vi "DCPower_ConfigureInstrument_V2.vi"(0 "IVI Refnum in":refnum<k15>, 1 "current limit":dbl, 2 "Aperture Time":dbl, 3 "Measure Record Length":i32, 4 "Active Channels Input":bool[](array[boolean]), 5 "Channel Name Array":string[](array[string]), 7 "error in (no error)":errorcluster, 8 "Voltage Array Input":dbl[](array[numeric]), 10 "DCPowerInformationClusterArray_Input":T1(array[cluster])) -> (12 "Active Channels Indicator":bool[](array[boolean]), 14 "All Channel Numbers Array":string[](array[string]), 16 "Total Voltage Indicator Array":dbl[](array[numeric]), 17 "All Channels Numbers List":string, 18 "Active Channel Numbers String List":string, 19 "IVI Ref index":i32, 20 "IVI Refnum out":refnum<k15>, 21 "Active Channel Numbers Array":string[](array[string]), 22 "Active Channel Names Array":string[](array[string]), 23 "Active Channel Current Limit Array":dbl[](array[numeric]), 24 "Active Channel Measure Record Delta Time Array":dbl[](array[numeric]), 25 "Active Channel Voltage Array":dbl[](array[numeric]), 26 "IVI Ref Present?":bool, 27 "error out":errorcluster)   [LabVIEW 2019]
panel:
  in  "DCPowerInformationClusterArray_Input_":T2(array[cluster])
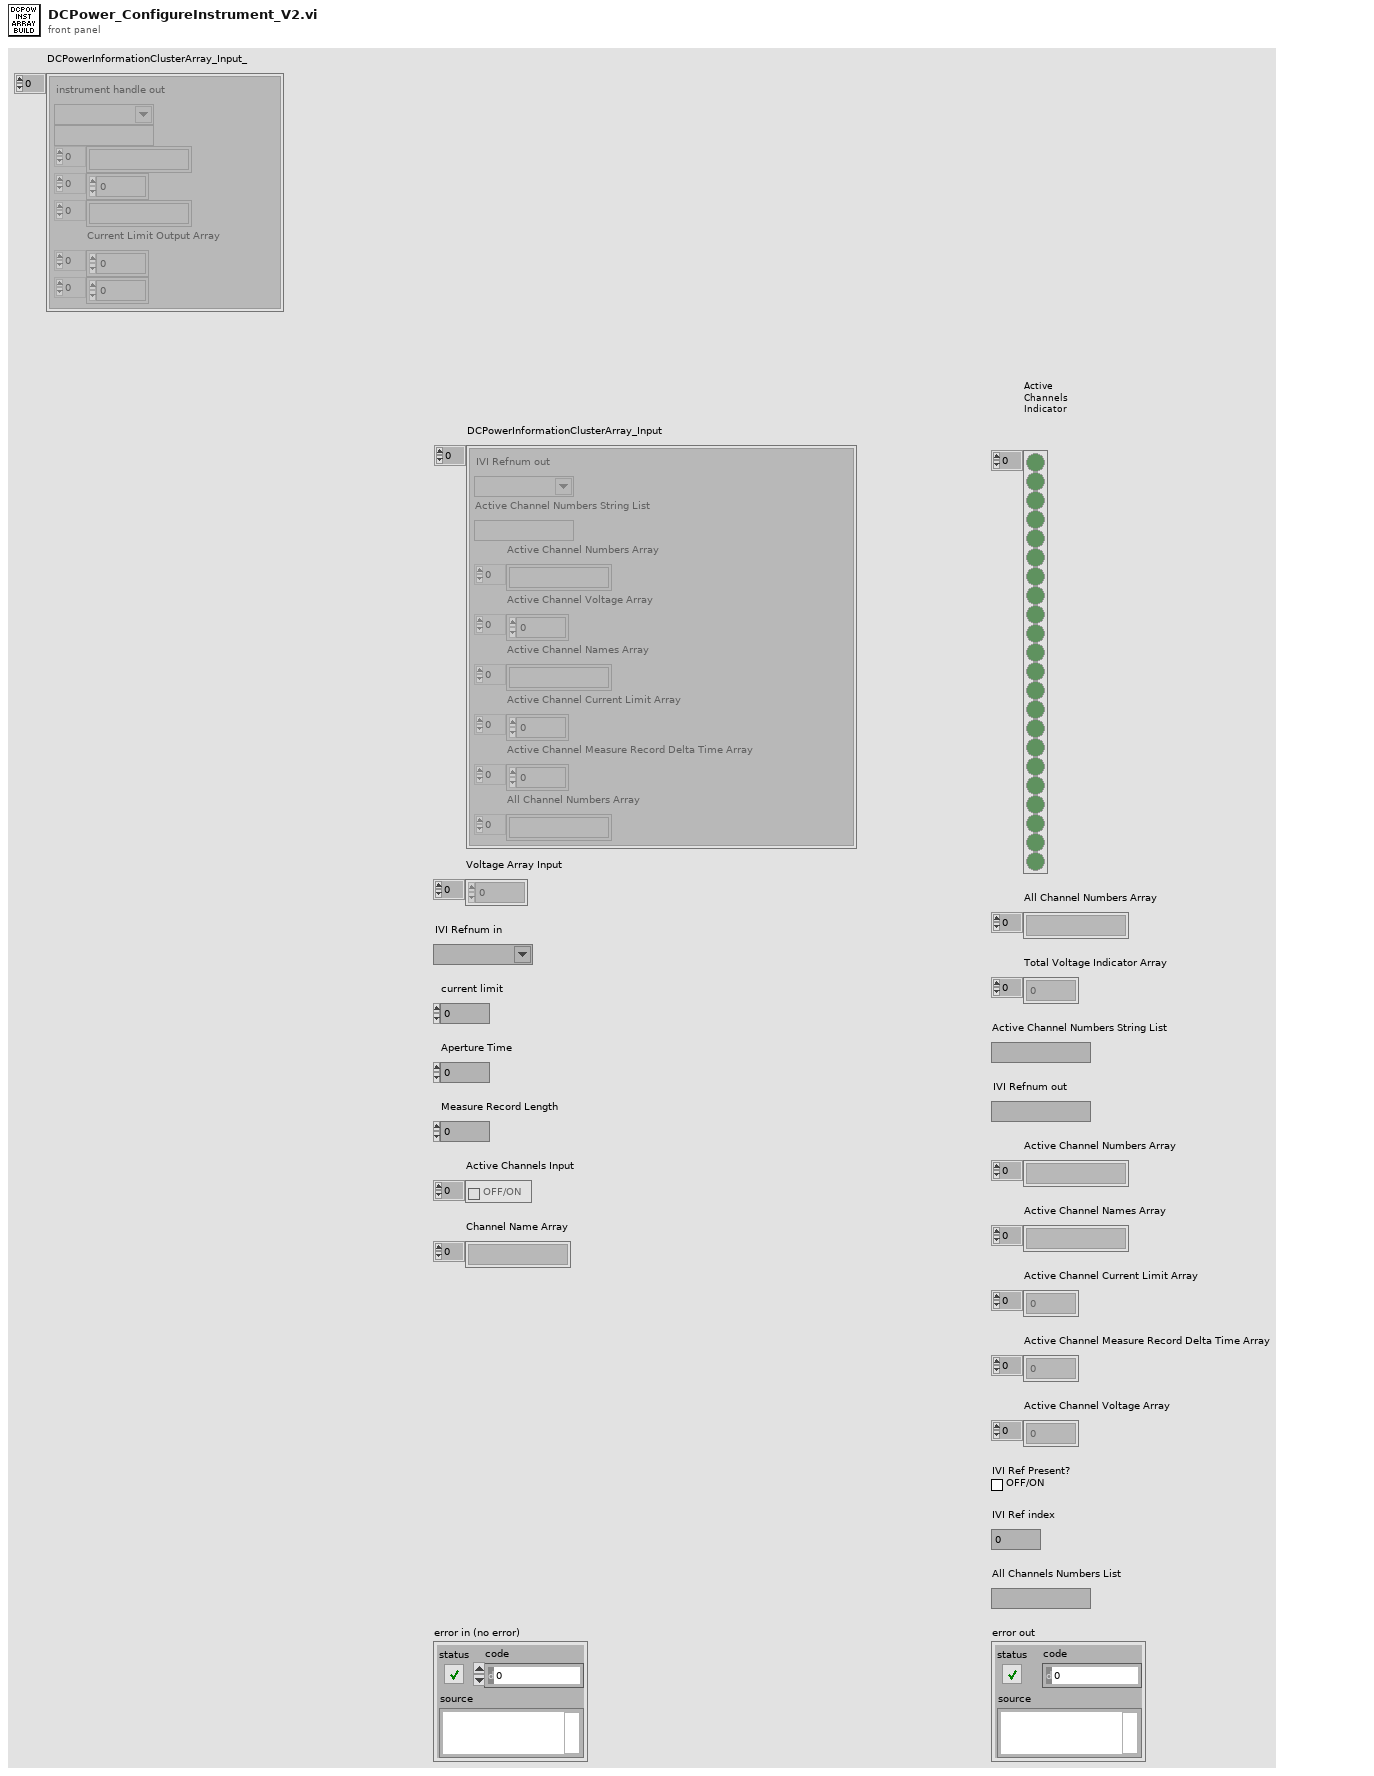
[diagram p1: front panel]
types:
  T1 = cluster{"IVI Refnum out":refnum<k15>, "Active Channel Numbers String List":string, "Active Channel Numbers Array":string[], "Active Channel Voltage Array":dbl[], "Active Channel Names Array":string[], "Active Channel Current Limit Array":dbl[], "Active Channel Measure Record Delta Time Array":dbl[], "All Channel Numbers Array":string[]}[]
  T2 = cluster{"instrument handle out":refnum<k15>, string, string[], dbl[], string[], "Current Limit Output Array":dbl[], dbl[]}[]
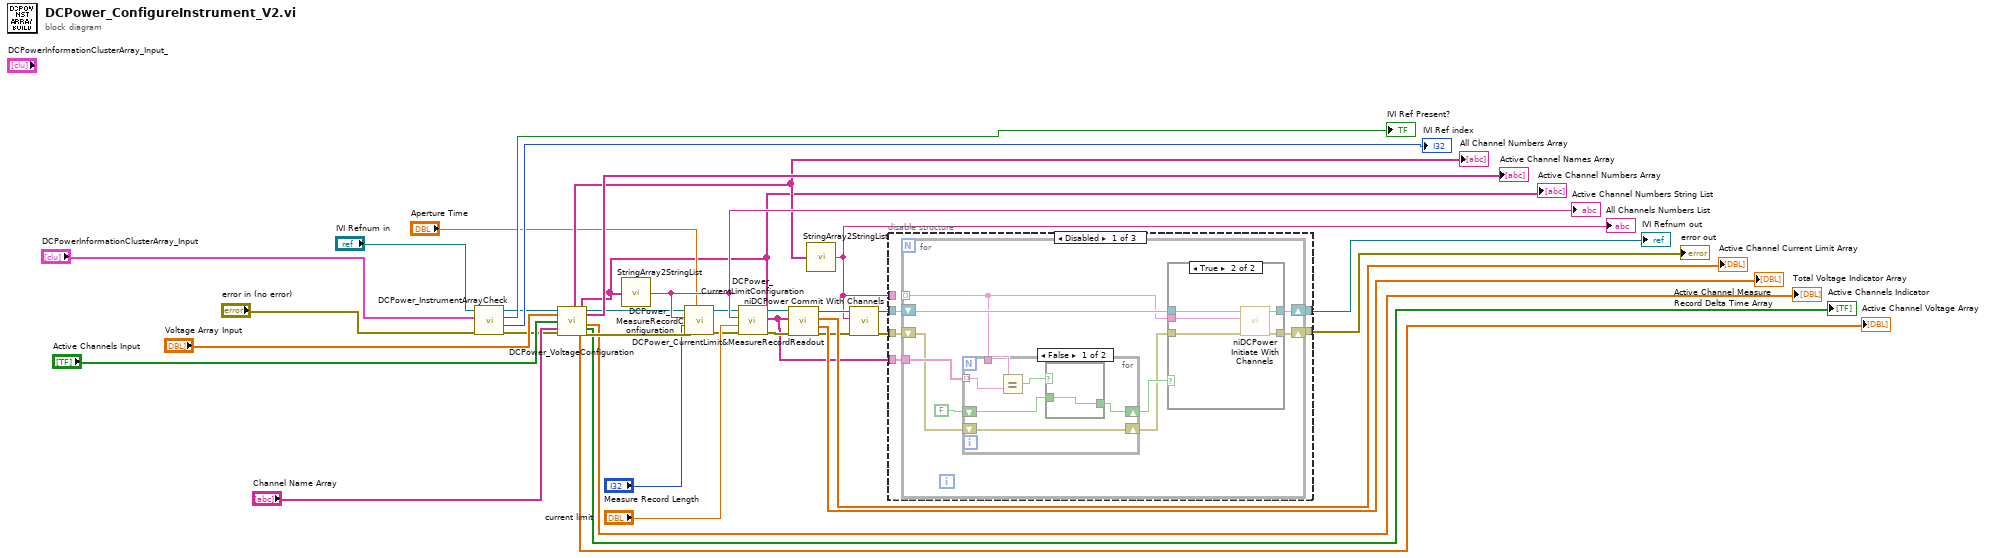
[diagram p0: block diagram]
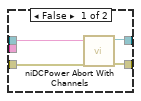
[diagram p2: hidden frame]
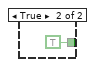
[diagram p3: hidden frame]
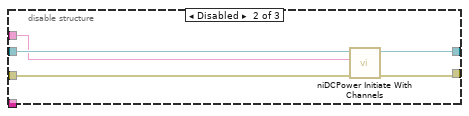
[diagram p4: hidden frame]
diagram:
  n1 = call "DCPower_InstrumentArrayCheck.vi"("error in (no error)"="error in (no error)", "DCPowerInformationClusterArray_Input"="DCPowerInformationClusterArray_Input", "IVI Refnum in"="IVI Refnum in") -> ("error out"=w9:errorcluster, "IVI Ref index"=→"IVI Ref index":i32, "IVI Ref Present?"=→"IVI Ref Present?":bool, "IVI Refnum out"=w8:refnum<k15>)  [unwired: 5 in]
  n2 = call "DCPower_VoltageConfiguration.vi"("IVI Refnum in"=w8, "Voltage Value By Channel"="Voltage Array Input", "Active Channels on Instrument"="Active Channels Input", "Channel Name Array"="Channel Name Array", "error in (no error)"=w9) -> ("All Channel Numbers Array"=w28:string[], "Active Channel Numbers Array"=w5:string[], "Active Channel Voltage Array"=→"Active Channel Voltage Array":dbl[], "IVI Refnum out"=w17:refnum<k15>, "Active Channel Names Array"=→"Active Channel Names Array":string[], "Total Voltage Indicator Array"=→"Total Voltage Indicator Array":dbl[], "Active Channels Indicator Array"=→"Active Channels Indicator":bool[], "error out"=w18:errorcluster)  [unwired: 7 in]
  "Active Channel Numbers Array" <- w5
  "All Channel Numbers Array" <- w28
  n3 = call "StringArray2StringList.vi"("String Array"=w5) -> ("String List"=w35:string)
  "Active Channel Numbers String List" <- w35
  n4 = call "DCPower_MeasureRecordConfiguration.vi"("Aperture Time"="Aperture Time", "error in (no error)"=w18, "Measure Record Length"="Measure Record Length", "Active Channel Numbers String"=w35, "IVI Refnum in"=w17) -> ("error out"=w20:errorcluster, "IVI Refnum out"=w19:refnum<k15>)  [unwired: 5 in]
  n5 = call "DCPower_CurrentLimitConfiguration.vi"("error in (no error)"=w20, "current limit"="current limit", "Active Channel Numbers String"=w35, "IVI Refnum in"=w19) -> ("error out"=w23:errorcluster, "IVI Refnum out"=w22:refnum<k15>)  [unwired: 6 in]
  n6 = call "DCPower_CurrentLimit&MeasureRecordReadout.vi"("error in (no error)"=w23, "Active Channel Numbers Array"=w5, "IVI Refnum in"=w22) -> ("error out"=w25:errorcluster, "Active Channel Measure Record Delta Time Array"=→"Active Channel Measure Record Delta Time Array":dbl[], "Active Channel Current Limit Array"=→"Active Channel Current Limit Array":dbl[], "IVI Refnum out"=w24:refnum<k15>)  [unwired: 5 in]
  n7 = call "StringArray2StringList.vi"("String Array"=w28) -> ("String List"=w4:string)
  "All Channels Numbers List" <- w4
  n8 = call <instrlib>:"niDCPower Commit With Channels.vi"("error in (no error)"=w25, "channel name"=w4, "instrument handle"=w24) -> ("error out"=w27:errorcluster, "instrument handle out"=w26:refnum<k15>)  [unwired: 7 in]
  n9 = disable-structure shown="Disabled" {
    disable-tunnel: w27 -> [w40 w69 w73]
    disable-tunnel: w26 -> [w39 w70 w74]
    disable-tunnel: w5 -> [w38 _ _]
    disable-tunnel: [w37 w72 w73] -> w2
    disable-tunnel: [w36 w71 w74] -> w3
    disable-tunnel: w4 -> [_ w68 _]
    frame Disabled {
      n10 = for {
        tunnel: _ -> [w45] mode=indexing
        shift-right: [w47] -> w37
        shift-left: w40 -> [w42]
        shift-right: [w48] -> w36
        shift-left: w39 -> [w49]
        tunnel: w38 -> [w46]
        n11 = for {
          tunnel: w46 -> [w64] mode=indexing
          tunnel: w45 -> [w65]
          shift-right: [w61] -> w44
          shift-left: FALSE -> [w62]
          shift-right: [w60] -> w41
          shift-left: w42 -> [w60]
          n12 = Equal?(x=w65, y=w64) -> (x = y?=w63:bool)
          n13 = case shown="False" w63 {
            tunnel: w62 -> [w66 _]
            tunnel: [w66 TRUE] -> w61
            frame False {
            }
            frame True {
            }
          }
        }
        n14 = case shown="True" w44 {
          tunnel: w49 -> [w50 w59]
          tunnel: w41 -> [w52 w58]
          tunnel: w45 -> [w51 w57]
          tunnel: [w54 w56] -> w48
          tunnel: [w53 w55] -> w47
          frame False {
            n15 = call <instrlib>:"niDCPower Abort With Channels.vi"("error in (no error)"=w52, "channel name"=w51, "instrument handle"=w50) -> ("error out"=w53:errorcluster, "instrument handle out"=w54:refnum<k15>)  [unwired: 7 in]
          }
          frame True {
            n16 = call <instrlib>:"niDCPower Initiate With Channels.vi"("error in (no error)"=w58, "channel name"=w57, "instrument handle"=w59) -> ("error out"=w55:errorcluster, "instrument handle out"=w56:refnum<k15>)  [unwired: 7 in]
          }
        }
      }
    }
    frame Disabled {
      n17 = call <instrlib>:"niDCPower Initiate With Channels.vi"("error in (no error)"=w69, "channel name"=w68, "instrument handle"=w70) -> ("error out"=w72:errorcluster, "instrument handle out"=w71:refnum<k15>)  [unwired: 7 in]
    }
    frame Enabled {
    }
  }
  "error out" <- w2
  "IVI Refnum out" <- w3
